vi "GetWorkingDirectoryEXEorSource.vi"(8 "ErrorIn":errorcluster) -> (0 "ErrorOut":errorcluster, 3 "Directory":path)   [LabVIEW 2018]
doc: "Return a path to the application operating directory. This directory varies depending on whether we are running this as a VI within the LabVIEW environment or as an EXE application with the LabVIEW runtime engine. \n\nUse this VI with caution as it may lead to unexpected changes in behavior when switching to EXE mode. In some cases, it may be advisable to instead use the File Constant VIs and treat the application directory the same whether running as a VI or EXE. \n\nCopyright © 2011 Epimedia, Inc. All Rights Reserved.\n\nThe Epimedia Application Library is Copyright © 2009-2011 Epimedia, Inc. \nAll Rights Reserved. Used under license."
panel:
  # "Copyright © 2011 Epimedia, Inc. All Rights Reserved.\n\nThe Epimedia Application Library is Copyright © 2009-2011 Epimedia, Inc. \nAll Rights Reserved. Used under license."
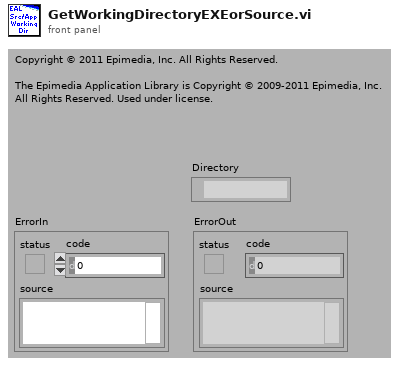
[diagram p1: front panel]
types:
  T1 = enum32{"invalid app kind", "Development System", "Run Time System", "Student Edition", "Embedded LabVIEW", "Evaluation", "Custom"}
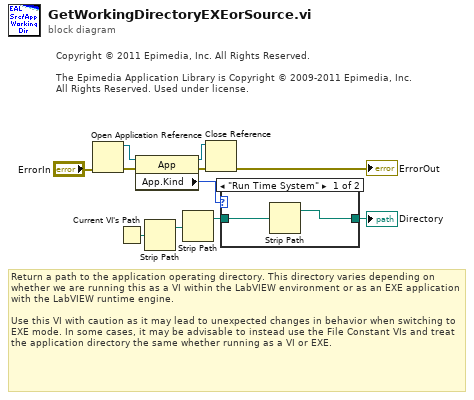
[diagram p0: block diagram]
diagram:
  # "Return a path to the application operating directory. This directory varies depending on whether we are running this as a VI within the LabVIEW environment or as an EXE application with the LabVIEW runtime engine.  \n\nUse this VI with caution as it may lead to unexpected changes in behavior when switching to EXE mode. In some cases, it may be advisable to instead use the File Constant VIs and treat the application directory the same whether running as a VI or EXE."
  # "Copyright © 2011 Epimedia, Inc. All Rights Reserved.\n\nThe Epimedia Application Library is Copyright © 2009-2011 Epimedia, Inc. \nAll Rights Reserved. Used under license."
  n1 = Open Application Reference(8:"ErrorIn") -> (0:w11:errorcluster, 3:w10:refnum<vi>)  [unwired: 3 out]
  n2 = Current VI's Path() -> (path=w5:path)
  n3 = property class="App"(reference=w10, error in=w11) -> (reference out=w8:refnum<vi>, error out=w9:errorcluster, "App.Kind"=w3:T1)
  n4 = Strip Path(path=w5) -> (stripped path=w6:path)  [unwired: 1 out]
  n5 = Strip Path(path=w6) -> (stripped path=w4:path)  [unwired: 1 out]
  n6 = Close Reference(reference=w8, error in (no error)=w9) -> (error out=→"ErrorOut":errorcluster)
  n7 = case shown="\"Run Time System\"" w3 {
    tunnel: [w13 w14] -> w7
    tunnel: w4 -> [w12 w14]
    frame "Run Time System" {
      n8 = Strip Path(path=w12) -> (stripped path=w13:path)  [unwired: 1 out]
    }
    frame Default {
    }
  }
  "Directory" <- w7
